vi "Write UUT Data.vi"(8 "error in (no error)":errorcluster, 10 "UUT Data (\"*IDN?\\r\\n\")":string="\"*IDN?\r\n\"", 11 "VISA resource name":refnum<visa-resource-name>) -> (0 "error out":errorcluster, 3 "VISA resource name out":refnum<visa-resource-name>)   [LabVIEW 2011, in "Fluke 5XXX Series Multicalibrators.lvlib"]
doc: "This VI sends data to the UUT serial port in binary block or string data format over the Calibrator rear panel SERIAL 2 TO UUT serial port. The command may be sent over gpib or RS-232 ports, but applies to SERIAL 2 TO UUT serial port operation. Include a line feed (RS-232) character to terminate the block data or End or Identify (EOI) command (IEEE-488).\n\nNote:\n\nThis VI is available only for instrument models 5500A and 5520A."
uses:
  Fluke 5XXX Series Multicalibrators.lvlib
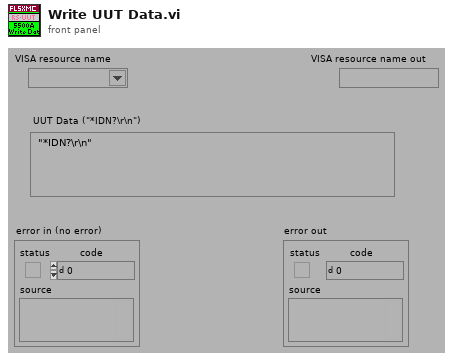
[diagram p1: front panel]
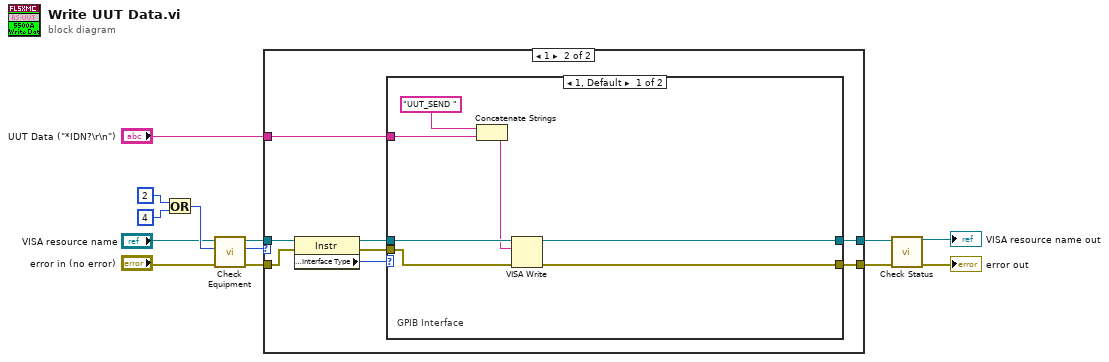
[diagram p0: block diagram]
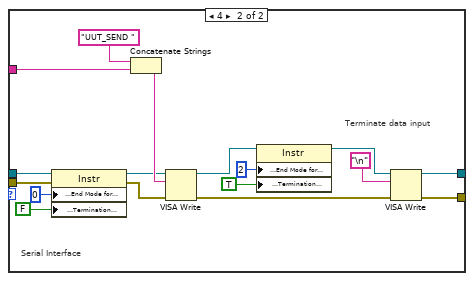
[diagram p3: hidden frame]
diagram:
  n1 = Or(x=u32 2, y=u32 4) -> (x .or. y?=w11:u32)
  n2 = call "Check Equipment.vi"("error in (no error)"="error in (no error)", "Bit Mask"=w11, "VISA resource name"="VISA resource name") -> ("error out"=w13:errorcluster, "Present?"=w8:u32, "VISA resource name out"=w12:refnum<visa-resource-name>)  [unwired: 6 in]
  n3 = case shown="1" w8 {
    tunnel: w13 -> [w14 w16]
    tunnel: w12 -> [w15 w17]
    tunnel: [w15 w19] -> w1
    tunnel: [w14 w18] -> w4
    tunnel: "UUT Data (\"*IDN?\\r\\n\")" -> [_ w20]
    frame 0, Default {
    }
    frame 1 {
      n4 = property class="Instr"(reference=w17, error in=w16) -> (reference out=w22:refnum<visa-resource-name>, error out=w21:errorcluster, "Interface Information:Interface Type"=w23:u16)
      n5 = case shown="1, Default" w23 {
        tunnel: w22 -> [w30 w43]
        tunnel: w21 -> [w28 w42]
        tunnel: w20 -> [w26 w37]
        tunnel: [w29 w35] -> w19
        tunnel: [w27 w34] -> w18
        frame 1, Default {
          # "GPIB Interface"
          n6 = Concatenate Strings("UUT_SEND " ("Substring"), w26) -> (w25:string)
          n7 = VISA Write(VISA resource name=w30, write buffer=w25, error in (no error)=w28) -> (VISA resource name out=w29:refnum<visa-resource-name>, error out=w27:errorcluster)  [unwired: 1 out]
        }
        frame 4 {
          # "Terminate data input"
          # "Serial Interface"
          n8 = property class="Instr"(reference=w43, error in=w42, "Serial Settings:End Mode for Writes"=u16 0 ("ASRL End In"), "Message Based Settings:Termination Character Enable"=FALSE ("TermChar En")) -> (reference out=w38:refnum<visa-resource-name>, error out=w39:errorcluster)
          n9 = Concatenate Strings("UUT_SEND " ("Substring"), w37) -> (w41:string)
          n10 = VISA Write(VISA resource name=w38, write buffer=w41, error in (no error)=w39) -> (VISA resource name out=w36:refnum<visa-resource-name>, error out=w32:errorcluster)  [unwired: 1 out]
          n11 = property class="Instr"(reference=w36, "Serial Settings:End Mode for Writes"=u16 2 ("ASRL End In"), "Message Based Settings:Termination Character Enable"=TRUE ("TermChar En")) -> (reference out=w33:refnum<visa-resource-name>)  [unwired: 1 in, 1 out]
          n12 = VISA Write(VISA resource name=w33, write buffer="\n" ("write buffer (\"\")"), error in (no error)=w32) -> (VISA resource name out=w35:refnum<visa-resource-name>, error out=w34:errorcluster)  [unwired: 1 out]
        }
      }
    }
  }
  n13 = call "Check Status.vi"("VISA resource name"=w1, "error in (no error)"=w4) -> ("VISA resource name out"=→"VISA resource name out":refnum<visa-resource-name>, "error out"=→"error out":errorcluster)  [unwired: 12 in]
